vi "flip.vi"(8 "error in (no error)":errorcluster, 10 "flip type":enum16{"Vertical", "Horizontal", "Both"}(ring), 11 "Image in":T1) -> (0 "error out":errorcluster, 3 "Image out":T1)   [LabVIEW 2024, in "Vision.lvlib"]
uses:
  Vision.lvlib
  <vilib>/vision/Image Controls.llb/IMAQ Image.ctl
  bin/Vision.dll
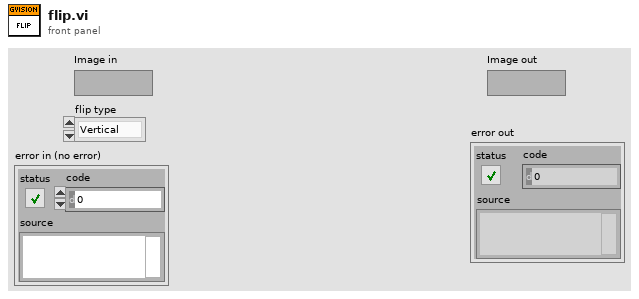
[diagram p1: front panel]
types:
  T1 = typedef "IMAQ Image.ctl" = refnum<image>
  T2 = enum32{"Map Pixel Pointer", "Unmap Pixel Pointer", "Get Pixels Infos"}
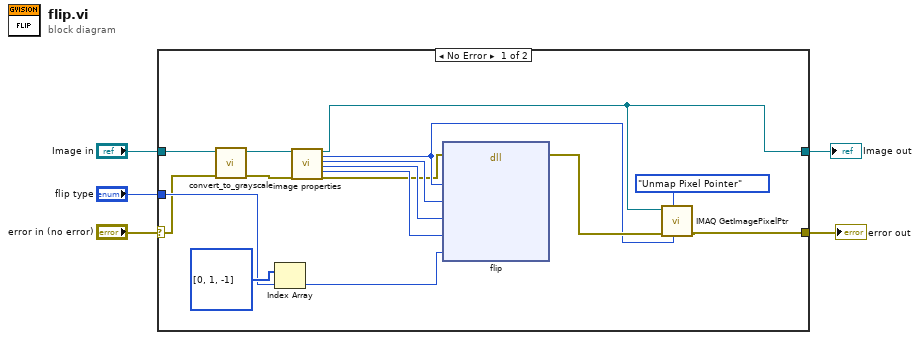
[diagram p0: block diagram]
diagram:
  n1 = case shown="No Error" "error in (no error)" {
    selector: "error in (no error)" -> [w6 w23]
    tunnel: "Image in" -> [w9 w22]
    tunnel: [w11 w23] -> w3
    tunnel: [w10 w22] -> w2
    tunnel: "flip type" -> [w13 _]
    frame No Error {
      n2 = call "convert_to_grayscale.vi"("error in (no error)"=w6, "Image in"=w9) -> ("error out"=w7:errorcluster, "Image out"=w8:T1)  [unwired: 8 in]
      n3 = Index Array(array=i32[] [0, 1, -1], index=w13) -> (element=w12:i32)
      n4 = call "image properties.vi"("Image in"=w8, "error in (no error)"=w7) -> ("Image out"=w10:T1, "Pixel Pointer out"=w19:u64, "Line Width"=w18:i32, "X Resolution"=w17:i32, "Y Resolution"=w16:i32, "error out"=w15:errorcluster)  [unwired: 10 in, 2 out]
      n5 = dll-call lib="C:/Users/cfang/Desktop/nebraska-silicon-lab/pixel-gantry-control/Gantry/Shared Components/bin/Vision.dll" fn="flip"(error in=w15, "src_imgPtr"=w19, "src_imgLineWidth"=w18, "src_imgWidth"=w17, "src_imgHeight"=w16, "flipType"=w12) -> (error out=w21:errorcluster)  [unwired: 8 in, 1 out]
      n6 = call "IMAQ GetImagePixelPtr"("Pixel Pointer in"=w19, "Function"=T2."Unmap Pixel Pointer", "error in (no error)"=w21, "Image"=w10) -> ("error out"=w11:errorcluster)  [unwired: 2 in, 5 out]
    }
    frame Error {
    }
  }
  "Image out" <- w2
  "error out" <- w3
